vi "Track Limelight Target.vi"() -> (2 "Joystick X":dbl)   [LabVIEW 2019]
uses:
  <vilib>/Rock Robotics/Network Tables/NT Read Number.vi
  <vilib>/addons/control/pid/pid.llb/PID (DBL).vi
  Robot Global Data.vi
  <vilib>/Rock Robotics/Network Tables/NT Write Number.vi
  <vilib>/addons/control/pid/NI_PID_pid.lvlib
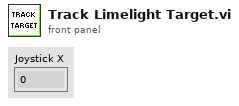
[diagram p1: front panel]
types:
  T1 = cluster{"proportional gain (Kc)":dbl, "integral time (Ti, min)":dbl, "derivative time (Td, min)":dbl}
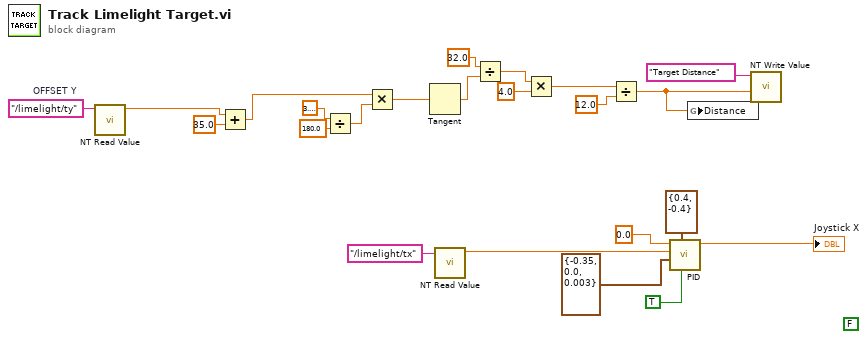
[diagram p0: block diagram]
diagram:
  (unwired) FALSE
  w7 = "/limelight/ty"  # OFFSET Y
  n1 = call-poly <vilib>:"NT Read Value.vi"("Name"=w7) -> ("Numeric"=w9:dbl)  [unwired: 9 in, 1 out]
  n2 = Add(x=w9, y=35.0) -> (x+y=w11:dbl)
  n3 = Divide(x=3.141592653589793, y=180.0) -> (x/y=w2:dbl)
  n4 = Multiply(x=w11, y=w2) -> (x*y=w3:dbl)
  n5 = Tangent(1:w3) -> (0:w4:dbl)
  n6 = call-poly <vilib>:"NT Read Value.vi"("Name"="/limelight/tx") -> ("Numeric"=w15:dbl)  [unwired: 9 in, 1 out]
  n7 = Divide(x=32.0, y=w4) -> (x/y=w12:dbl)
  n8 = Multiply(x=w12, y=4.0) -> (x*y=w21:dbl)
  n9 = Divide(x=w21, y=12.0) -> (x/y=w22:dbl)
  n10 = call-poly <vilib>:"PID.vi"("reinitialize? (F)"=TRUE, "output range"=cluster{"output high":dbl, "output low":dbl} {"output high"=0.4, "output low"=-0.4}, "PID gains"=T1 {"proportional gain (Kc)"=-0.35, "integral time (Ti, min)"=0.0, "derivative time (Td, min)"=0.003}, "process variable"=w15, "setpoint"=0.0) -> ("output"=→"Joystick X":dbl)  [unwired: 5 in, 1 out]
  n11 = global write "Robot Global Data.vi" "Distance"(w22) -> ()
  n12 = call-poly <vilib>:"NT Write Value.vi"("Numeric"=w22, "Name"="Target Distance") -> ()  [unwired: 9 in, 1 out]
